vi "Factorial.vi"() -> ()   [LabVIEW 2019]
panel:
  out "Factorial":i32
  in  "Numeric":i32
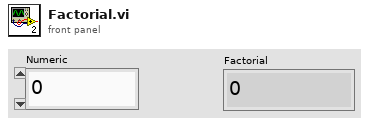
[diagram p1: front panel]
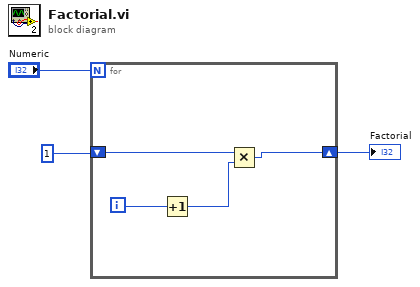
[diagram p0: block diagram]
diagram:
  n1 = for {
    N: "Numeric" -> [_]
    shift-right: [w6] -> w1
    shift-left: 1 -> [w7]
    i -> [w5]
    n2 = Increment(x=w5) -> (x+1=w4:i32)
    n3 = Multiply(x=w7, y=w4) -> (x*y=w6:i32)
  }
  "Factorial" <- w1
